vi "Update Add Run Subpanel.vi"(8 "error in (no error)":errorcluster, 11 "Optimiser SBlock in":refnum<class "Optimiser SBlock.lvclass">) -> (0 "error out":errorcluster, 2 "reference out":refnum<vi>, 3 "Optimiser SBlock out":refnum<class "Optimiser SBlock.lvclass">)   [LabVIEW 2020, in "CIRCUS_uServices.lvlib" / "Run Utilities.lvlib" / "Optimiser SBlock.lvclass"]
uses:
  Optimiser SBlock.lvclass
  Optimiser SBlock.lvclass/Optimiser SBlock.ctl
  Optimiser Mode Panel.vi
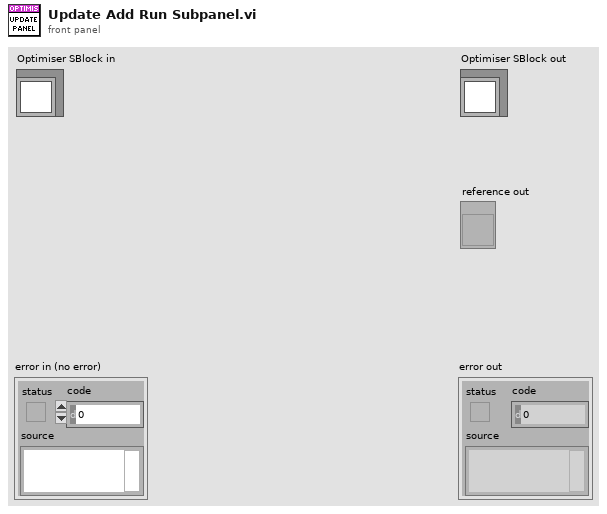
[diagram p1: front panel]
types:
  T1 = typedef "CIRCUS_uServices.lvlib/Run Utilities.lvlib/Optimiser Cell.lvclass/Optimisation Strategy.ctl" = enum16{"Maximize", "Minimize", "Value"}
  T2 = typedef "CIRCUS_uServices.lvlib/Run Utilities.lvlib/Optimiser Cell.lvclass/Optimise parameter - numeric.ctl" = cluster{"Name":string, "Start value":dbl, "From":dbl, "To":dbl, "dtype":enum16{"INT", "DBL"}}
  T3 = typedef "CIRCUS_uServices.lvlib/Run Utilities.lvlib/Optimiser Cell.lvclass/Optimise parameter - string.ctl" = cluster{"Name":string, "Start value":string, "Options":string[]}
  T4 = typedef "CIRCUS_uServices.lvlib/Run Utilities.lvlib/Optimiser Cell.lvclass/Optimisation observable.ctl" = cluster{"Name":string, "Weight":dbl}
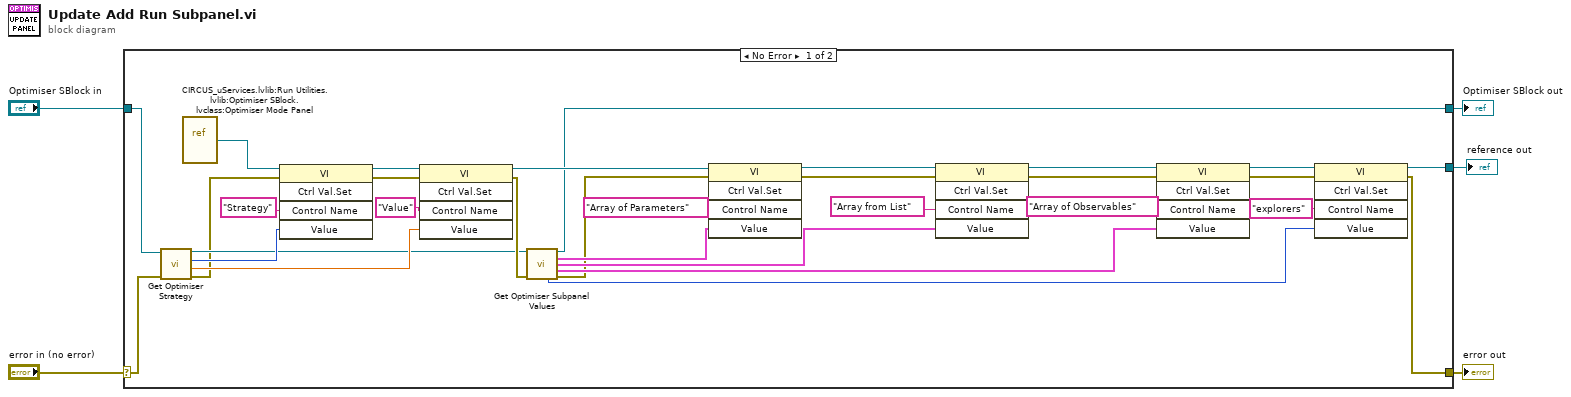
[diagram p0: block diagram]
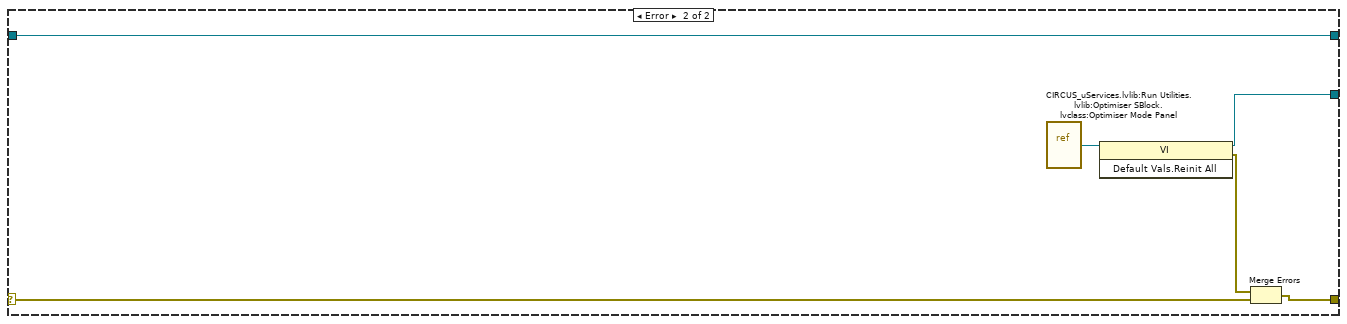
[diagram p2: hidden frame]
diagram:
  n1 = case shown="No Error" "error in (no error)" {
    selector: "error in (no error)" -> [w8 w38]
    tunnel: [w6 w37] -> w4
    tunnel: [w7 w42] -> w2
    tunnel: "Optimiser SBlock in" -> [w10 w42]
    tunnel: [w9 w40] -> w1
    frame No Error {
      n2 = call-dynamic "Get Optimiser Strategy.vi"("error in (no error)"=w8, "Optimiser SBlock in"=w10) -> ("error out"=w17:errorcluster, "Value"=w34:dbl, "Optimisation Strategy"=w35:T1, "Optimiser SBlock out"=w29:refnum<class "Optimiser SBlock.lvclass">)  [unwired: 6 in]
      n3 = vi-ref "CIRCUS_uServices.lvlib:Run Utilities.lvlib:Optimiser SBlock.lvclass:Optimiser Mode Panel.vi"() -> (w36:refnum<vi>)
      n4 = invoke class="VI" method="Ctrl Val.Set"(reference=w36, error in=w17, "Control Name"="Strategy", "Value"=w35) -> (reference out=w32:refnum<vi>, error out=w33:errorcluster)  [unwired: 1 in, 3 out]
      n5 = invoke class="VI" method="Ctrl Val.Set"(reference=w32, error in=w33, "Control Name"="Value", "Value"=w34) -> (reference out=w31:refnum<vi>, error out=w30:errorcluster)  [unwired: 1 in, 3 out]
      n6 = call "Get Optimiser Subpanel Values.vi"("Optimiser SBlock in"=w29, "error in (no error)"=w30) -> ("Optimiser SBlock out"=w7:refnum<class "Optimiser SBlock.lvclass">, "Parameters - Numeric"=w21:T2[], "Parameters - String"=w28:T3[], "Observables"=w22:T4[], "Number of Exploration Runs"=w23:i32, "error out"=w20:errorcluster)  [unwired: 8 in]
      n7 = invoke class="VI" method="Ctrl Val.Set"(reference=w31, error in=w20, "Control Name"="Array of Parameters", "Value"=w21) -> (reference out=w24:refnum<vi>, error out=w26:errorcluster)  [unwired: 1 in, 3 out]
      n8 = invoke class="VI" method="Ctrl Val.Set"(reference=w24, error in=w26, "Control Name"="Array from List", "Value"=w28) -> (reference out=w25:refnum<vi>, error out=w27:errorcluster)  [unwired: 1 in, 3 out]
      n9 = invoke class="VI" method="Ctrl Val.Set"(reference=w25, error in=w27, "Control Name"="Array of Observables", "Value"=w22) -> (reference out=w18:refnum<vi>, error out=w19:errorcluster)  [unwired: 1 in, 3 out]
      n10 = invoke class="VI" method="Ctrl Val.Set"(reference=w18, error in=w19, "Control Name"="explorers", "Value"=w23) -> (reference out=w9:refnum<vi>, error out=w6:errorcluster)  [unwired: 1 in, 3 out]
    }
    frame Error {
      n11 = vi-ref "CIRCUS_uServices.lvlib:Run Utilities.lvlib:Optimiser SBlock.lvclass:Optimiser Mode Panel.vi"() -> (w41:refnum<vi>)
      n12 = invoke class="VI" method="Default Vals.Reinit All"(reference=w41) -> (reference out=w40:refnum<vi>, error out=w39:errorcluster)  [unwired: 2 in, 1 out]
      n13 = Merge Errors(w39, w38) -> (w37:errorcluster)
    }
  }
  "error out" <- w4
  "Optimiser SBlock out" <- w2
  "reference out" <- w1
